vi "Discovery.vi"(8 "Error In":errorcluster caption="error out", 9 "ShowMess":bool) -> (0 "error out":errorcluster, 3 "IP":string)   [LabVIEW 2019]
panel:
  # "This VI checks for all connected AMCs in your network. \nYou can use it instead of manually or statically assigning an IP address to the \"AMC_connect\" VI.\n \nIn case no devices can be found a warning message appears.\nin case only one AMC is connected, its IP gets automatically chosen. \nIn case more than one AMC is connected a \"select IP pop-up\" will appear."
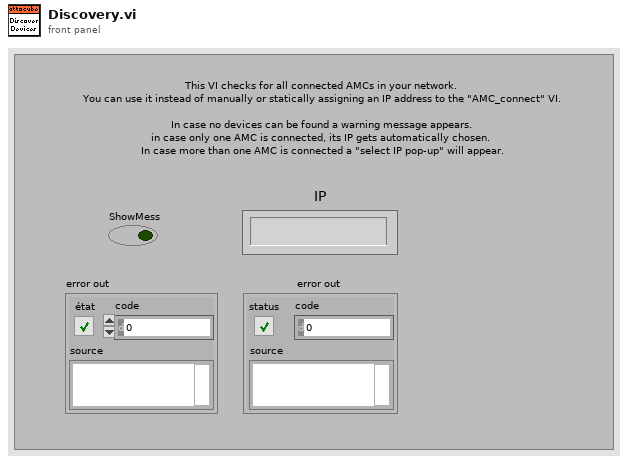
[diagram p1: front panel]
types:
  T1 = cluster{"IP":string, "DeviceType":string, "SerialNumber":string, "DeviceName":string, "macAddress":string, "locked":bool}[]
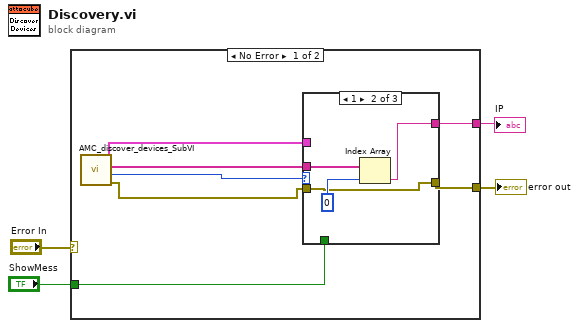
[diagram p0: block diagram]
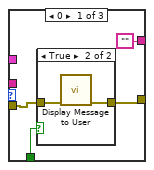
[diagram p2: hidden frame]
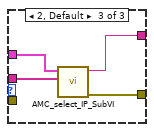
[diagram p4: hidden frame]
diagram:
  n1 = case shown="No Error" "Error In" {
    tunnel: [w8 _] -> w4
    tunnel: [w7 _] -> w3
    tunnel: "ShowMess" -> [w6 _]
    frame No Error {
      n2 = call "AMC_discover_devices_SubVI.vi"() -> ("error out"=w5:errorcluster, "No. of found devices"=w9:i32, "IPs"=w10:string[], "Found Devices"=w11:T1)  [unwired: 8 in]
      n3 = case shown="1" w9 {
        tunnel: w11 -> [_ _ w26]
        tunnel: w10 -> [_ w21 w25]
        tunnel: ["" w20 w24] -> w7
        tunnel: [w14 w19 w23] -> w8
        tunnel: w5 -> [w13 w19 _]
        tunnel: w6 -> [w12 _ _]
        frame 0 {
          n4 = case shown="True" w12 {
            tunnel: [w16 w18] -> w14
            tunnel: w13 -> [w16 w17]
            frame False {
            }
            frame True {
              n5 = call "Display Message to User"("error in (no error)"=w17) -> ("error out"=w18:errorcluster)  [unwired: 9 in, 1 out]
            }
          }
        }
        frame 1 {
          n6 = Index Array(array=w21, index=0) -> (element=w20:string)
        }
        frame 2, Default {
          n7 = call "AMC_select_IP_SubVI.vi"("IPs"=w25, "Found Devices"=w26) -> ("error out"=w23:errorcluster, "IP"=w24:string)  [unwired: 7 in, 1 out]
        }
      }
    }
    frame Error {
    }
  }
  "IP" <- w3
  "error out" <- w4
